vi "XY_Graph.vi"(1 "a":enum16{""}[](array[ring]), 2 "x":dbl[](array[numeric])) -> (0 "XY Graph":cluster{i32[], dbl[]}[](graph))   [LabVIEW 2015]
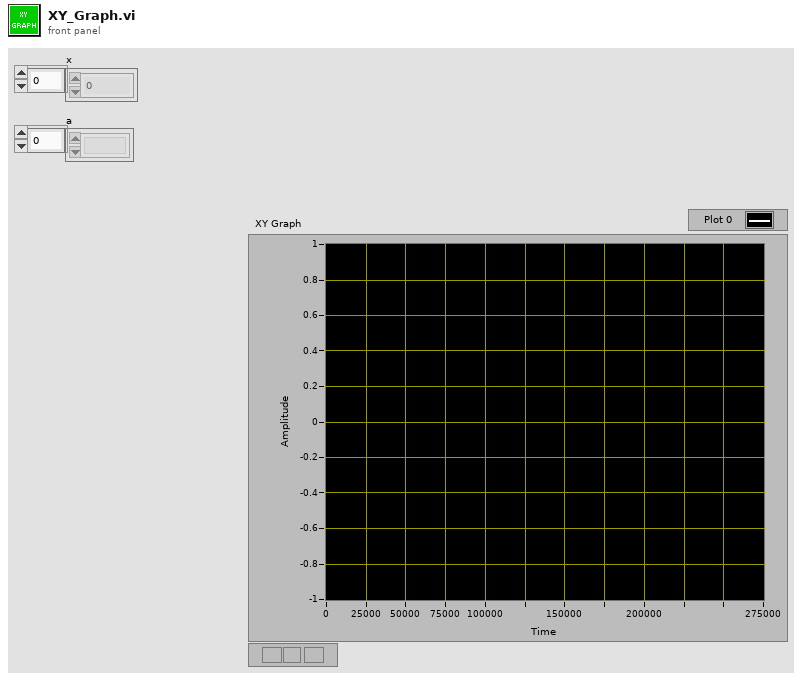
[diagram p1: front panel]
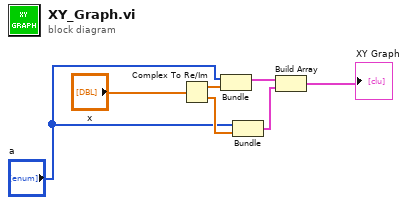
[diagram p0: block diagram]
diagram:
  n1 = Complex To Re/Im(x + iy="x") -> (x=w7:dbl[], y=w6:dbl[])
  n2 = Bundle("a"="a", w7) -> (w5:cluster{"a":enum16{""}[], dbl[]})  [unwired: 1 in]
  n3 = Bundle("a"="a", w6) -> (w4:cluster{"a":enum16{""}[], dbl[]})  [unwired: 1 in]
  n4 = Build Array(w5, w4) -> (→"XY Graph":cluster{"a":enum16{""}[], dbl[]}[])
